vi "Speech Recognition - Main.vi"() -> ()   [LabVIEW 2012]
uses:
  <vilib>/NXT/Block Support/NXT_OutputPort.ctl
  <vilib>/NXT/NXT Controls/ConnectionType.ctl
panel:
  out "Time":u32
  out "Boolean":bool
  out "Score":dbl
  in  "Phrases":i32(listbox)
  in  "Exit":bool
  out "Command":string
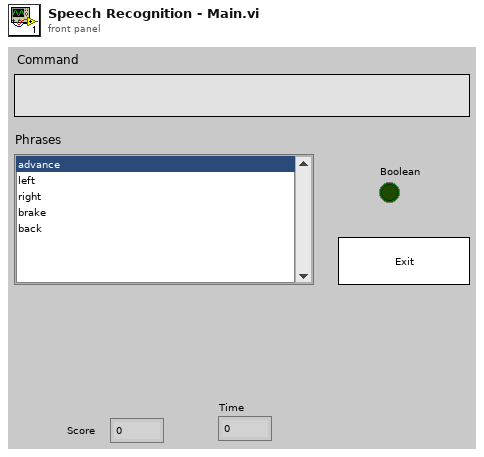
[diagram p1: front panel]
types:
  T1 = typedef "ConnectionType.ctl" = enum16{"Bluetooth", "USB"}
  T2 = typedef "nxt.ctl" = cluster{"nxtHandle":u32, "fileHandle":u32, "fileIterHandle":u32, "moduleHandle":u32, "modIterHandle":u32, "nxtIterHandle":u32}
  T3 = typedef "NXT_OutputPort.ctl" = u8
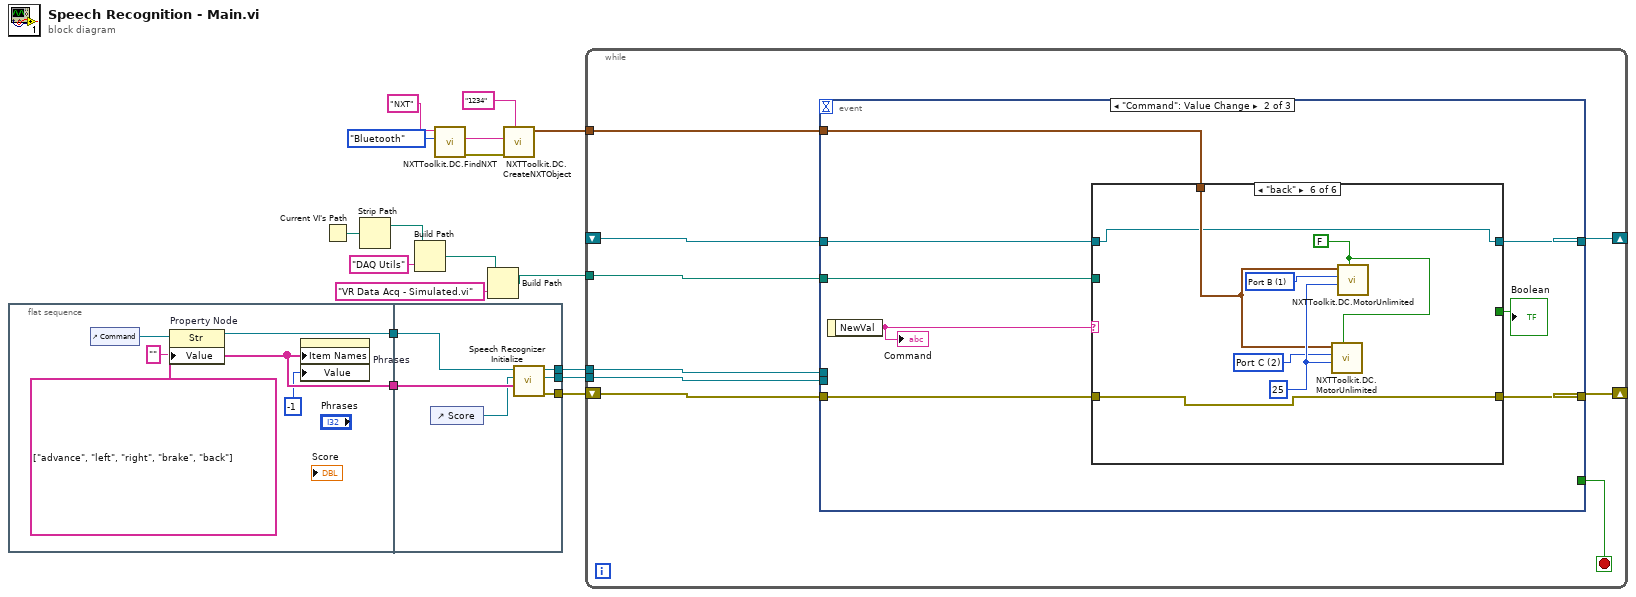
[diagram p0: block diagram]
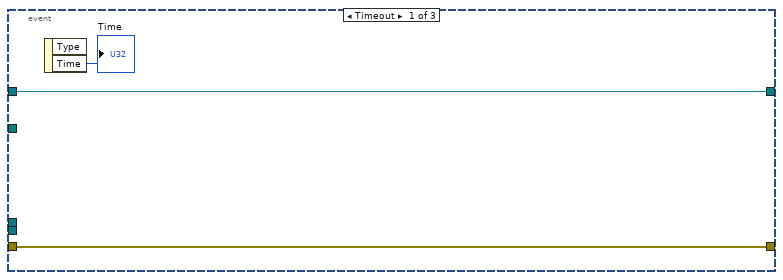
[diagram p2: hidden frame]
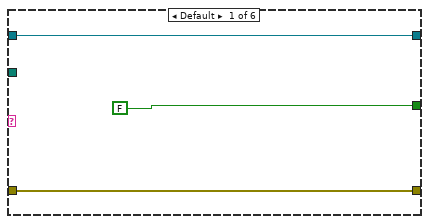
[diagram p3: hidden frame]
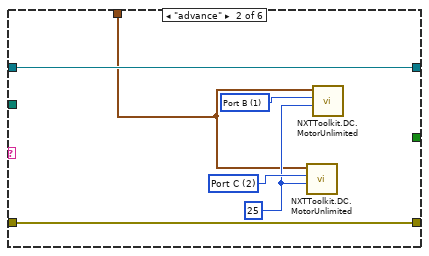
[diagram p4: hidden frame]
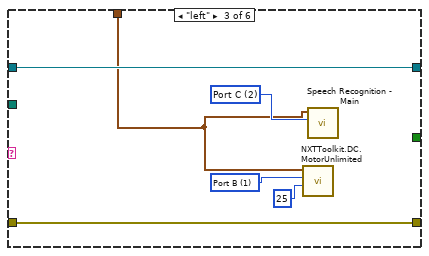
[diagram p5: hidden frame]
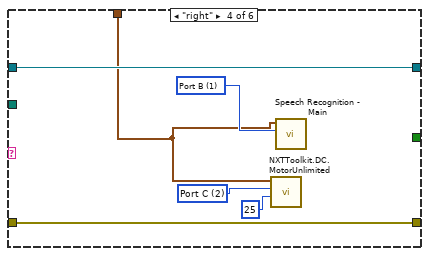
[diagram p6: hidden frame]
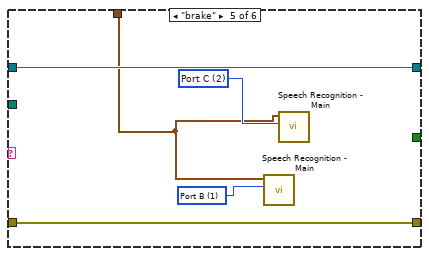
[diagram p7: hidden frame]
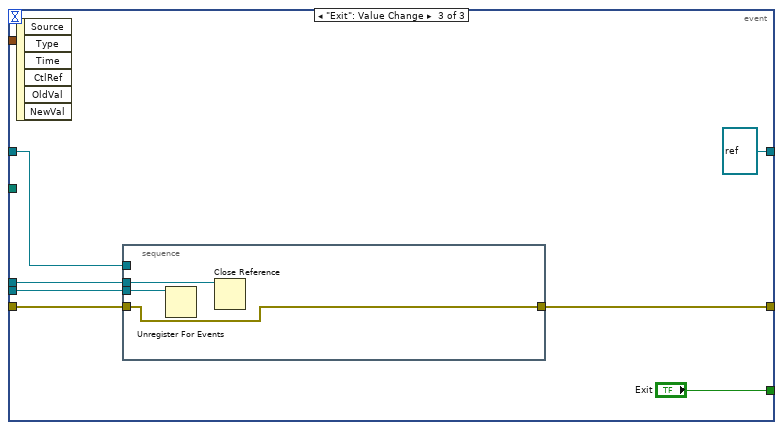
[diagram p8: hidden frame]
diagram:
  n1 = flat-sequence {
    tunnel: [w22] -> w14
    tunnel: [w19] -> w7
    tunnel: [w28] -> w17
    tunnel: [w27] -> w16
    tunnel: [w26] -> w15
    tunnel: w14 -> [w25]
    tunnel: w7 -> [w23]
    frame #0 {
      w22 = string[] ["advance", "left", "right", "brake", "back"] ("Item Names")
      n2 = control-ref of="Command"() -> (w21:refnum<vi>)
      n3 = property on="Property Node" class="Str"(reference=w21, "Value"="") -> (reference out=w19:refnum<vi>)  [unwired: 1 in, 1 out]
      n4 = property on="Phrases" class="LstBox (strict)"("Item Names"=w22, "Value"=-1) -> ()  [unwired: 2 in, 2 out]
    }
    frame #1 {
      n5 = control-ref of="Score"() -> (w24:refnum<vi>)
      n6 = call "Speech Recognizer Initialize.vi"("String[] phrases"=w25, "Score"=w24, "Text"=w23) -> ("error out"=w28:errorcluster, "Event Callback"=w27:refnum<k27>, "reference"=w26:refnum<k24>)  [unwired: 6 in]
    }
  }
  n7 = Current VI's Path() -> (path=w9:path)
  n8 = Strip Path(path=w9) -> (stripped path=w8:path)  [unwired: 1 out]
  n9 = Build Path(base path=w8, name or relative path="DAQ Utils") -> (appended path=w12:path)
  n10 = call <vilib>:"NXTToolkit.DC.FindNXT.vi"("Connection type (USB)"=ConnectionType."Bluetooth", "NXT name"="NXT") -> ("error out"=w2:errorcluster, "VISA resource string"=w3:string)  [unwired: 7 in, 1 out]
  n11 = Build Path(base path=w12, name or relative path="VR Data Acq - Simulated.vi") -> (appended path=w10:path)
  n12 = call <vilib>:"NXTToolkit.DC.CreateNXTObject.vi"("Bluetooth passkey (1234)"="1234", "error in (no error)"=w2, "VISA resource string (\"\" : find USB brick)"=w3) -> ("NXTObject"=w1:T2)  [unwired: 6 in, 2 out]
  n13 = while {
    shift-right: [w35] -> _
    shift-left: w17 -> [w37]
    tunnel: w16 -> [w34]
    tunnel: w15 -> [w33]
    tunnel: w10 -> [w32]
    shift-right: [w31] -> _
    shift-left: _ -> [w30]
    tunnel: w1 -> [w29]
    stop <- w36 stop-if-true
    n14 = event shown="[1] \"Command\": Value Change" {
      selector: _ -> [_ _ _]
      dyn-events: _ -> [_ _ _]
      timeout: _ -> [_ _ _]
      tunnel: w37 -> [w40 w48 w87]
      tunnel: [_ _ "Exit"] -> w36
      tunnel: [w40 w47 w82] -> w35
      tunnel: w34 -> [_ _ w86]
      tunnel: w33 -> [_ _ w85]
      tunnel: w32 -> [_ w45 _]
      tunnel: [w39 w44 refnum<vi> refnum ("vi reference")] -> w31
      tunnel: w30 -> [w39 w43 w84]
      tunnel: w29 -> [_ w41 _]
      event Timeout {
        n15 = event-data() -> ("Time"=→"Time":u32)  [unwired: 2 out]
      }
      event "Command": Value Change {
        n16 = event-data() -> ("NewVal"=w46:string)  [unwired: 1 out]
        "Command" <- w46
        n17 = case shown="\"back\"" w46 {
          tunnel: w48 -> [w51 w56 w62 w68 w73 w75]
          tunnel: [w51 w56 w62 w68 w73 w75] -> w47
          tunnel: w45 -> [_ _ _ _ _ _]
          tunnel: [w50 w57 w63 w69 w74 w76] -> w44
          tunnel: w43 -> [w50 w57 w63 w69 w74 w76]
          tunnel: [FALSE ("Boolean") _ _ _ _ _] -> w42
          tunnel: w41 -> [_ w52 w58 w64 w70 w78]
          frame Default {
          }
          frame "advance" {
            w54 = T3 2 items=["Port A", "Port B", "Port C"] ("Output Port (Port A)")
            w53 = i8 25 ("Power (75)")
            w55 = T3 1 items=["Port A", "Port B", "Port C"] ("Output Port (Port A)")
            n18 = call <vilib>:"NXTToolkit.DC.MotorUnlimited.vi"("Power (75)"=w53, "Output Port (Port A)"=w54, "NXTObject"=w52) -> ()  [unwired: 7 in, 2 out]
            n19 = call <vilib>:"NXTToolkit.DC.MotorUnlimited.vi"("Power (75)"=w53, "Output Port (Port A)"=w55, "NXTObject"=w52) -> ()  [unwired: 7 in, 2 out]
          }
          frame "left" {
            w59 = T3 1 items=["Port A", "Port B", "Port C"] ("Output Port (Port A)")
            w61 = T3 2 items=["Port A", "Port B", "Port C"] ("Output Port (Port A)")
            n20 = call <vilib>:"NXTToolkit.DC.MotorUnlimited.vi"("Power (75)"=i8 25, "Output Port (Port A)"=w59, "NXTObject"=w58) -> ()  [unwired: 7 in, 2 out]
            n21 = call "Speech Recognition - Main.vi"("Output Port (Port A)"=w61, "NXTObject"=w58) -> ()  [unwired: 8 in, 2 out]
          }
          frame "right" {
            w65 = T3 2 items=["Port A", "Port B", "Port C"] ("Output Port (Port A)")
            w67 = T3 1 items=["Port A", "Port B", "Port C"] ("Output Port (Port A)")
            n22 = call <vilib>:"NXTToolkit.DC.MotorUnlimited.vi"("Power (75)"=i8 25, "Output Port (Port A)"=w65, "NXTObject"=w64) -> ()  [unwired: 7 in, 2 out]
            n23 = call "Speech Recognition - Main.vi"("Output Port (Port A)"=w67, "NXTObject"=w64) -> ()  [unwired: 8 in, 2 out]
          }
          frame "brake" {
            w71 = T3 1 items=["Port A", "Port B", "Port C"] ("Output Port (Port A)")
            w72 = T3 2 items=["Port A", "Port B", "Port C"] ("Output Port (Port A)")
            n24 = call "Speech Recognition - Main.vi"("Output Port (Port A)"=w71, "NXTObject"=w70) -> ()  [unwired: 8 in, 2 out]
            n25 = call "Speech Recognition - Main.vi"("Output Port (Port A)"=w72, "NXTObject"=w70) -> ()  [unwired: 8 in, 2 out]
          }
          frame "back" {
            w77 = FALSE ("Direction (T: Fwd)")
            w80 = T3 2 items=["Port A", "Port B", "Port C"] ("Output Port (Port A)")
            w81 = i8 25 ("Power (75)")
            w79 = T3 1 items=["Port A", "Port B", "Port C"] ("Output Port (Port A)")
            n26 = call <vilib>:"NXTToolkit.DC.MotorUnlimited.vi"("Direction (T: Fwd)"=w77, "Power (75)"=w81, "Output Port (Port A)"=w80, "NXTObject"=w78) -> ()  [unwired: 6 in, 2 out]
            n27 = call <vilib>:"NXTToolkit.DC.MotorUnlimited.vi"("Direction (T: Fwd)"=w77, "Power (75)"=w81, "Output Port (Port A)"=w79, "NXTObject"=w78) -> ()  [unwired: 6 in, 2 out]
          }
        }
        "Boolean" <- w42
      }
      event "Exit": Value Change {
        n28 = event-data() -> ()  [unwired: 7 out]
        n29 = stacked-sequence {
          tunnel: w87 -> [w89]
          tunnel: w86 -> [w91]
          tunnel: w85 -> [w90]
          tunnel: w84 -> [_]
          tunnel: [w89] -> w82
          frame #0 {
            n30 = Unregister For Events(event registration refnum=w91) -> ()  [unwired: 1 in, 1 out]
            n31 = Close Reference(reference=w90) -> ()  [unwired: 1 in, 1 out]
          }
        }
      }
    }
  }
